vi "NI VeriStand - Get Target Operating System.vi"(8 "error in (no error)":errorcluster, 11 "Item Ref in":T1 format="%.0x") -> (0 "error out":errorcluster, 2 "Operating System Name":string, 3 "Item Ref out":T1 format="%.0x")   [LabVIEW 2026, in "SEECD System Explorer.lvlib"]
uses:
  SEECD System Explorer.lvlib
  <vilib>/NI VeriStand/Custom Device API/Custom Device Item Ref.ctl
  C:/Users/Administrator/Desktop/Jatin/All DNC DLLs/NationalInstruments.VeriStand.SystemDefinitionAPI.dll
  Jatin/All DNC DLLs/NationalInstruments.VeriStand.SystemDefinitionAPI.dll
  C:/Users/Administrator/Desktop/Jatin/All DNC DLLs/NationalInstruments.VeriStand.SystemStorage.dll
  Jatin/All DNC DLLs/NationalInstruments.VeriStand.SystemStorage.dll
  <vilib>/NI VeriStand/Custom Device Tools/Custom Device Utility Library/Custom Device Utility Library.lvlib
  <vilib>/NI VeriStand/Custom Device API/Custom Device API.lvlib
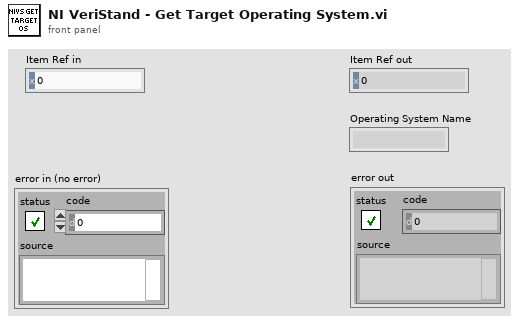
[diagram p1: front panel]
types:
  T1 = typedef "Custom Device API.lvlib/Custom Device Item Ref.ctl" = u64
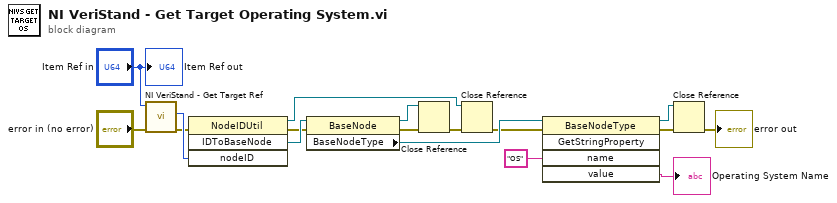
[diagram p0: block diagram]
diagram:
  n1 = call <vilib>:"NI VeriStand - Get Target Ref.vi"("error in"="error in (no error)", "Item Ref in"="Item Ref in") -> ("error out"=w3:errorcluster, "Target Ref"=w4:T1)  [unwired: 6 in, 2 out]
  n2 = invoke class="NodeIDUtil" method="IDToBaseNode"(error in=w3, "nodeID"=w4) -> (reference out=w8:refnum<k39>, error out=w9:errorcluster, "IDToBaseNode"=w10:refnum<k39>)  [unwired: 2 in, 1 out]
  n3 = property class="BaseNode"(reference=w10, error in=w9) -> (reference out=w6:refnum<k39>, error out=w7:errorcluster, "BaseNodeType"=w2:refnum<k39>)
  n4 = Close Reference(reference=w6, error in (no error)=w7) -> (error out=w5:errorcluster)
  n5 = Close Reference(reference=w8, error in (no error)=w5) -> (error out=w1:errorcluster)
  n6 = invoke class="BaseNodeType" method="GetStringProperty"(reference=w2, error in=w1, "name"="OS") -> (reference out=w17:refnum<k39>, error out=w16:errorcluster, "value"=→"Operating System Name":string)  [unwired: 2 in, 2 out]
  n7 = Close Reference(reference=w17, error in (no error)=w16) -> (error out=→"error out":errorcluster)
  "Item Ref out" <- "Item Ref in"
